vi "Open License Manager.vi"   [LabVIEW 2018]
doc: "Demonstrates how to activate a license through opening VIRobotics License Manager interface."
panel:
  # "Overview: Demonstrates how to activate a license through opening VIRobotics License Manager interface\nRequirements: Windows.\nInstructions: \n1.Run the VI"
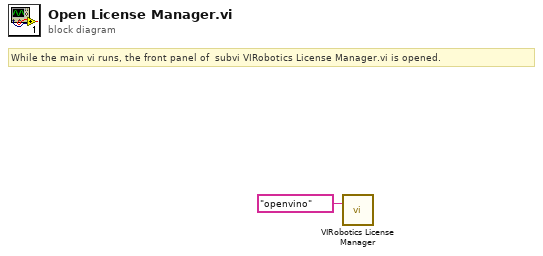
[diagram p0: block diagram]
diagram:
  # "While the main vi runs, the front panel of  subvi VIRobotics License Manager.vi is opened."
  n1 = call "VIRobotics License Manager.vi"("Product Name"="openvino") -> ()  [unwired: 11 in]
